vi "post_psu.vi"(8 "error in (no error)":errorcluster, 11 "PSU settings":T1={"Integer Timestamp"=0, "Max Velocity"=0.0, "Min Velocity"=0.0, "Max Charge"=0.0, "Min Charge"=0.0, "Max Mass"=0.0, "Min Mass"=0.0, "Variable 1"=enum."Mass", "Variable 2"=enum."Mass"}) -> (0 "error out":errorcluster)   [LabVIEW 2013]
doc: "Adds a new row to the dcs_spot table."
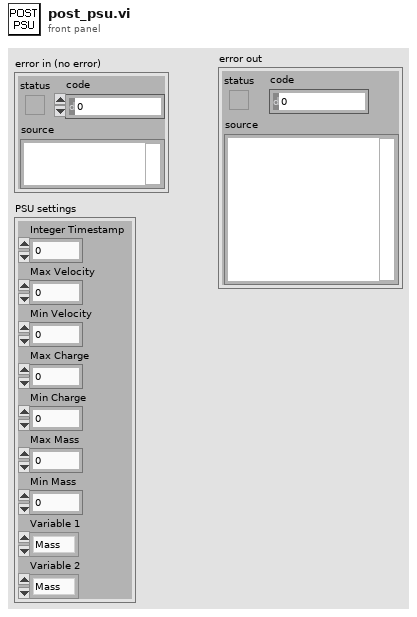
[diagram p1: front panel]
types:
  T1 = cluster{"Integer Timestamp":i64, "Max Velocity":dbl, "Min Velocity":dbl, "Max Charge":dbl, "Min Charge":dbl, "Max Mass":dbl, "Min Mass":dbl, "Variable 1":enum8{"Velocity", "Charge", "Mass"}, "Variable 2":enum8{"Velocity", "Charge", "Mass"}}
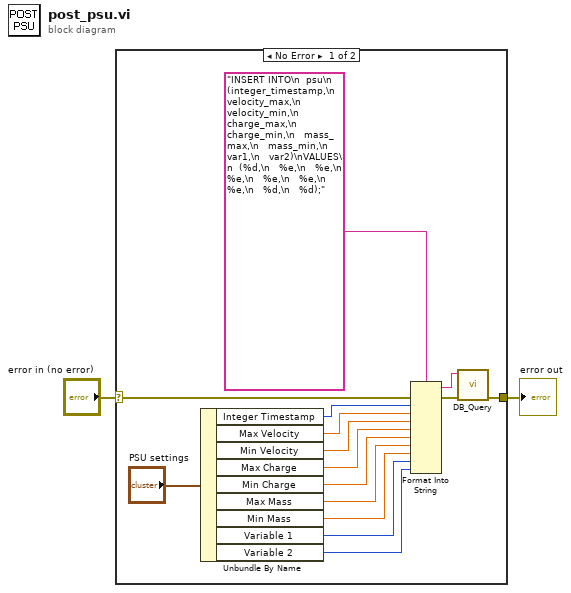
[diagram p0: block diagram]
diagram:
  n1 = case shown="No Error" "error in (no error)" {
    selector: "error in (no error)" -> [w17 w18]
    tunnel: [w10 w18] -> w1
    frame No Error {
      n2 = Unbundle By Name("PSU settings") -> ("Integer Timestamp"=w14:i64, "Max Velocity"=w13:dbl, "Min Velocity"=w12:dbl, "Max Charge"=w8:dbl, "Min Charge"=w7:dbl, "Max Mass"=w6:dbl, "Min Mass"=w5:dbl, "Variable 1"=w4:enum8{"Velocity", "Charge", "Mass"}, "Variable 2"=w3:enum8{"Velocity", "Charge", "Mass"})
      n3 = Format Into String(format string="INSERT INTO\n  psu\n  (integer_timestamp,\n   velocity_max,\n   velocity_min,\n   charge_max,\n   charge_min,\n   mass_max,\n   mass_min,\n   var1,\n   var2)\nVALUES\n  (%d,\n   %e,\n   %e,\n   %e,\n   %e,\n   %e,\n   %e,\n   %d,\n   %d);" ("Parameterized Query"), error in=w17, w14, w13, w12, w8, w7, w6, w5, w4, w3) -> (resulting string=w11:string, error out=w16:errorcluster)  [unwired: 1 in]
      n4 = call "DB_Query.vi"("error in (no error)"=w16, "Parameterized Query"=w11) -> ("error out"=w10:errorcluster)  [unwired: 7 in, 2 out]
    }
    frame Error {
    }
  }
  "error out" <- w1
